vi "PopulateQuizArrayfromFile.vi"(8 "error in (no error)":errorcluster, 11 "file path (dialog if empty)":path) -> (0 "error out":errorcluster, 1 "Raw Data":string[][](array[string]), 2 "Question Array Out":T1[](array[typedef]))   [LabVIEW 2010]
uses:
  Controls/Quiz Set Up.ctl
  Controls/Problem Type enum.ctl
  Controls/Solution Type enum.ctl
  <vilib>/Utility/file.llb/Read From Spreadsheet File (string).vi
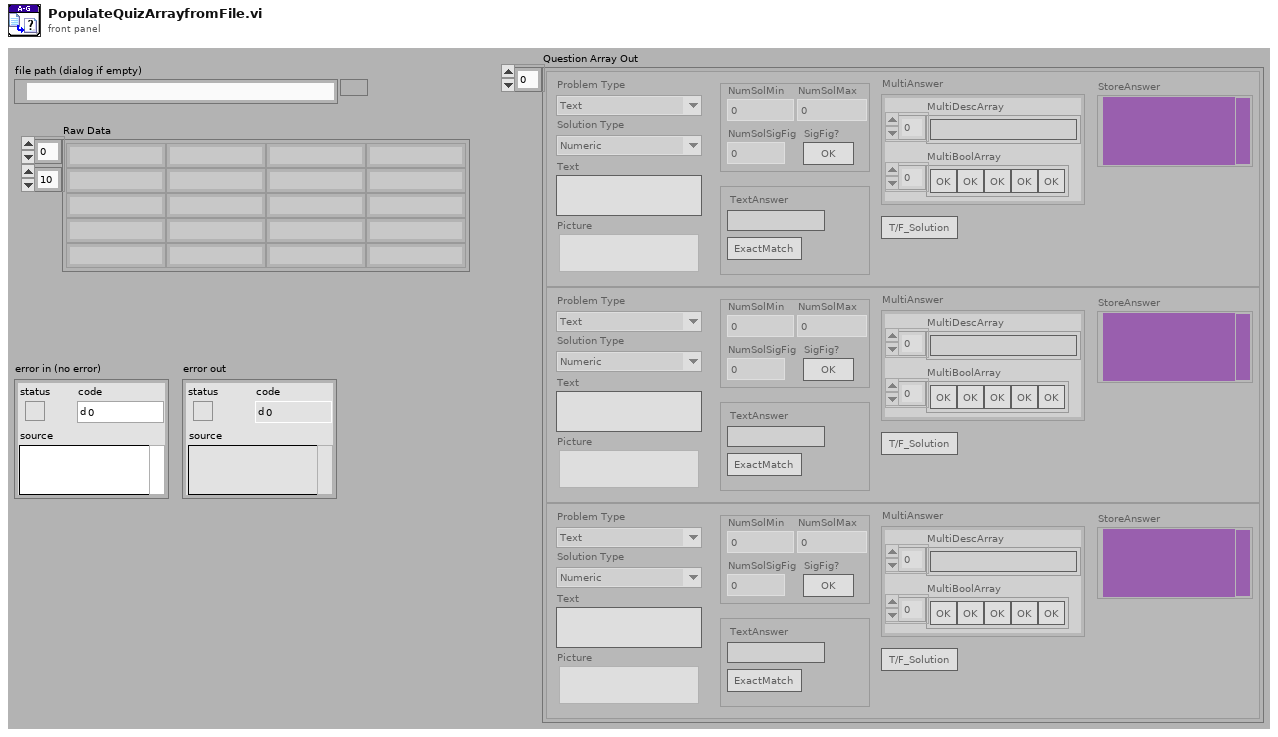
[diagram p1: front panel]
types:
  T1 = typedef "Quiz Set Up.ctl" = cluster{"Problem Type":T2, "Solution Type":T3, "Text":string, "Picture":picture, "NumSolMin":dbl, "NumSolMax":dbl, "SigFig?":bool, "NumSolSigFig":u32, "TextAnswer":string, "ExactMatch":bool, "T/F_Solution":bool, "StoreAnswer":variant, "MultiAnswer":cluster{"MultiDescArray":string[], "MultiBoolArray":bool[]}}
  T2 = typedef "Problem Type enum.ctl" = enum16{"Text", "Image", "Text&Image"}
  T3 = typedef "Solution Type enum.ctl" = enum16{"Numeric", "Text", "SelectMultiple", "SelectOne", "True/False", "ShortAnswer"}
  T4 = typedef "imagedata.ctl" = cluster{"image type":i32, "image depth":i32, "image":u8[], "mask":u8[], "colors":u32[], "Rectangle":cluster{"left":i16, "top":i16, "right":i16, "bottom":i16}}
  T5 = cluster{"MultiDescArray":string[], "MultiBoolArray":bool[]}
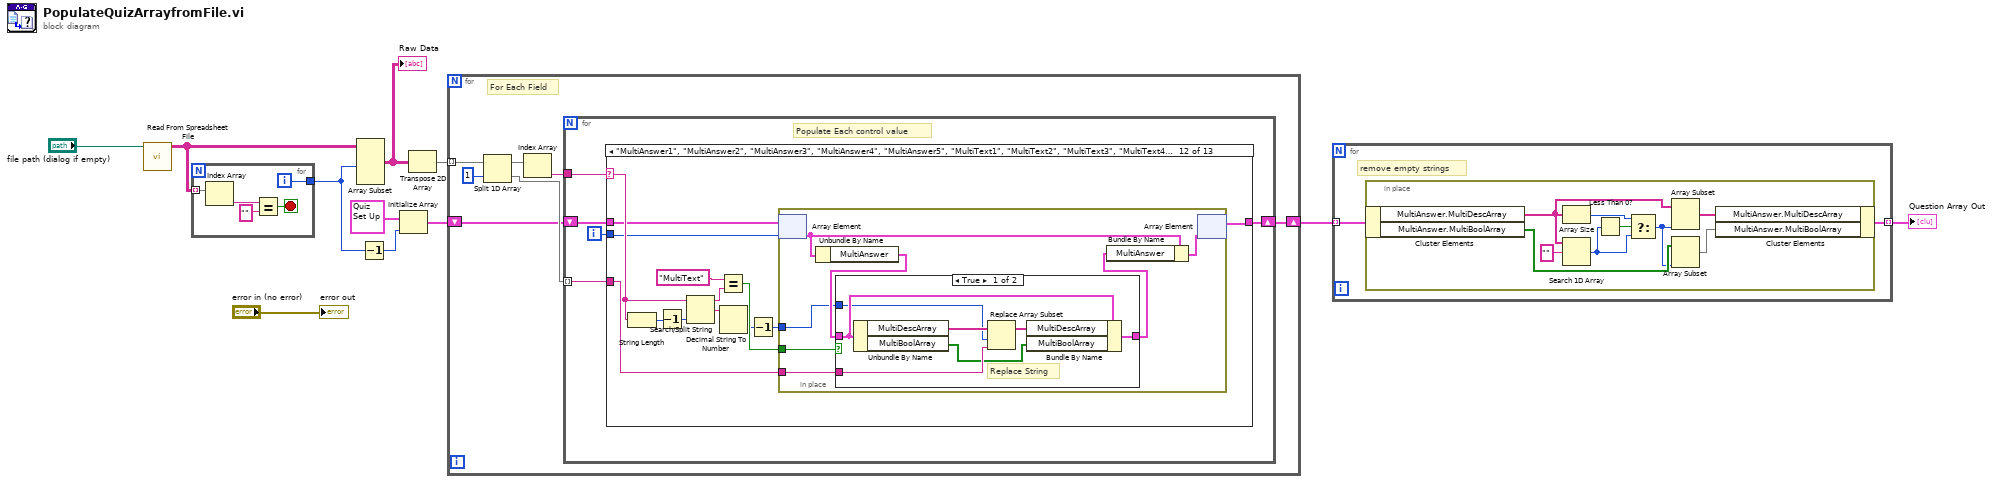
[diagram p0: block diagram]
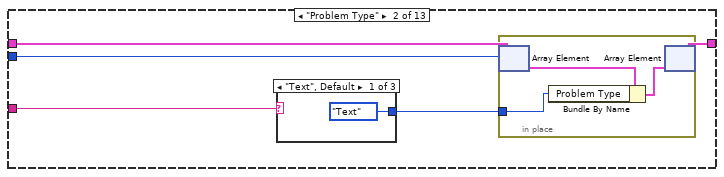
[diagram p3: hidden frame]
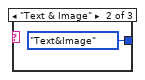
[diagram p4: hidden frame]
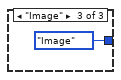
[diagram p5: hidden frame]
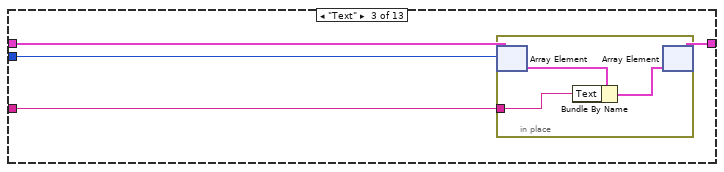
[diagram p6: hidden frame]
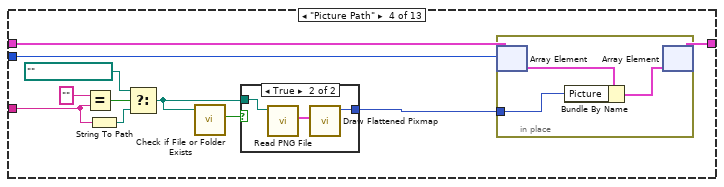
[diagram p7: hidden frame]
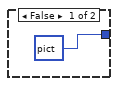
[diagram p8: hidden frame]
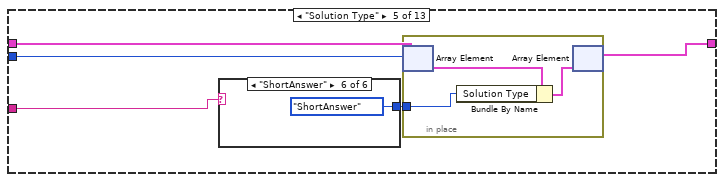
[diagram p9: hidden frame]
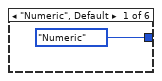
[diagram p10: hidden frame]
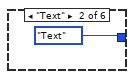
[diagram p11: hidden frame]
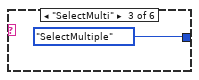
[diagram p12: hidden frame]
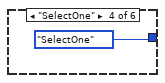
[diagram p13: hidden frame]
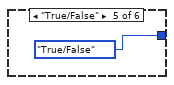
[diagram p14: hidden frame]
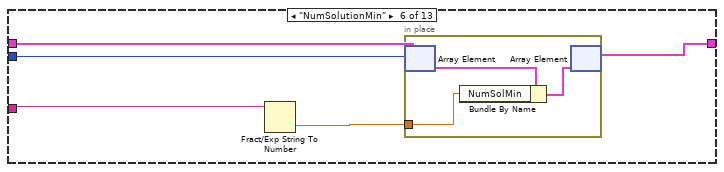
[diagram p15: hidden frame]
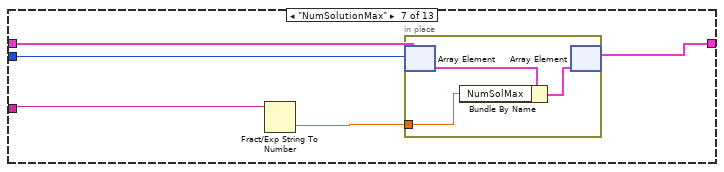
[diagram p16: hidden frame]
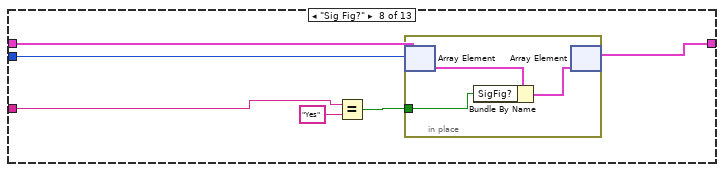
[diagram p17: hidden frame]
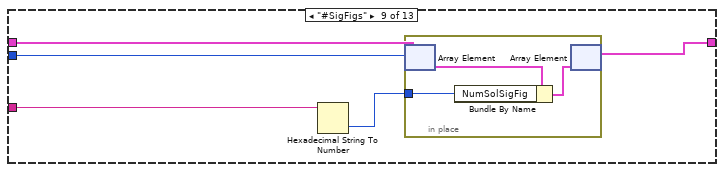
[diagram p18: hidden frame]
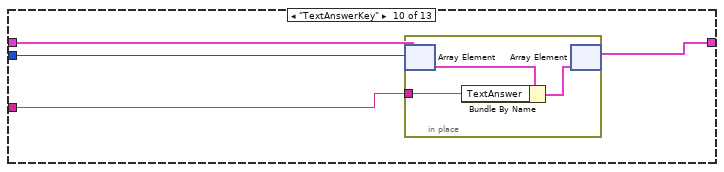
[diagram p19: hidden frame]
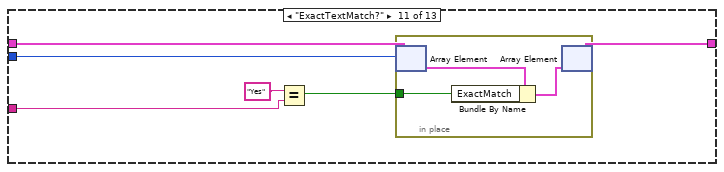
[diagram p20: hidden frame]
diagram:
  n1 = call-poly <vilib>:"Read From Spreadsheet File.vi"("file path (dialog if empty)"="file path (dialog if empty)") -> ("all rows"=w8:string[][])  [unwired: 6 in, 4 out]
  n2 = for {
    tunnel: [w15] -> w1
    tunnel: w8 -> [w14] mode=indexing
    i -> [w15]
    stop <- w12 stop-if-true
    n3 = Index Array(array=w14) -> (element=w13:string)  [unwired: 1 in]
    n4 = Equal?(x=w13, y="") -> (x = y?=w12:bool)
  }
  n5 = Array Subset(array=w8, length (row)=w1) -> (w9:string[][])  [unwired: 3 in]
  "Raw Data" <- w9
  n6 = Decrement(x=w1) -> (x-1=w2:i32)
  n7 = Initialize Array(T1 {"Problem Type"=enum."Text", "Solution Type"=enum."Numeric", "Text"="The sky is blue.", "Picture"=bytes[0], "NumSolMin"=0.0, "NumSolMax"=0.0, "SigFig?"=FALSE, "NumSolSigFig"=0, "TextAnswer"="", "ExactMatch"=FALSE, "T/F_Solution"=FALSE, "StoreAnswer"=variant, "MultiAnswer"={"MultiDescArray"=["", "", "", "", ""], "MultiBoolArray"=[FALSE, FALSE, FALSE, FALSE, FALSE]}} ("Quiz Set Up"), w2) -> (w5:T1[])
  n8 = Transpose 2D Array(2D array=w9) -> (transposed array=w11:string[][])
  n9 = for {
    tunnel: w11 -> [w23] mode=indexing
    shift-right: [w17] -> w3
    shift-left: w5 -> [w19]
    # "For Each Field"
    n10 = Split 1D Array(array=w23, index=1) -> (first subarray=w20:string[], second subarray=w21:string[])
    n11 = Index Array(array=w20) -> (element=w18:string)  [unwired: 1 in]
    n12 = for {
      tunnel: w21 -> [w28] mode=indexing
      tunnel: w18 -> [w27]
      shift-right: [w25] -> w17
      shift-left: w19 -> [w26]
      i -> [w24]
      # "Populate Each control value"
      n13 = case shown="\"MultiAnswer1\", \"MultiAnswer2\", \"MultiAnswer3\", \"MultiAnswer4\", \"MultiAnswer5\", \"MultiText1\", \"MultiText2\", \"MultiText3\", \"MultiText4\", \"MultiText5\"" w27 {
        selector: w27 -> [_ _ _ _ _ _ _ _ _ _ _ w136 _]
        tunnel: w28 -> [_ w34 w41 w53 w68 w84 w92 w98 w106 w113 w122 w130 w167]
        tunnel: w26 -> [w29 w33 w44 w57 w70 w82 w90 w100 w108 w115 w124 w135 w169]
        tunnel: [w29 w32 w43 w58 w69 w80 w88 w99 w107 w114 w125 w129 w170] -> w25
        tunnel: w24 -> [_ w30 w42 w55 w66 w83 w91 w101 w109 w116 w123 w134 w168]
        frame "NULL", Default {
        }
        frame "Problem Type" {
          n14 = case shown="\"Text\", Default" w34 {
            tunnel: [Problem_Type_enum."Text" ("Problem Type") Problem_Type_enum."Text&Image" ("Problem Type") Problem_Type_enum."Image" ("Problem Type")] -> w31
            frame "Text", Default {
            }
            frame "Text & Image" {
            }
            frame "Image" {
            }
          }
          n15 = in-place {
            in-place-border: w31 -> [w35]
            n16 = in-place-array #1(w33, w30) -> (w37:T1)
            n17 = Bundle By Name(cluster=w37, "Problem Type"=w35) -> (w36:T1)
            n18 = in-place-array #1(w36) -> (w32:T1[])  [unwired: 1 out]
          }
        }
        frame "Text" {
          n19 = in-place {
            in-place-border: w41 -> [w45]
            n20 = in-place-array #2(w44, w42) -> (w47:T1)
            n21 = Bundle By Name(cluster=w47, "Text"=w45) -> (w46:T1)
            n22 = in-place-array #2(w46) -> (w43:T1[])  [unwired: 1 out]
          }
        }
        frame "Picture Path" {
          n23 = Equal?(x="", y=w53) -> (x = y?=w51:bool)
          n24 = String To Path(string=w53) -> (path=w50:path)
          n25 = Select(t=path "", s=w51, f=w50) -> (s? t:f=w49:path)
          n26 = call <vilib>:"Check if File or Folder Exists.vi"("path"=w49) -> ("file or folder exists?"=w54:bool)  [unwired: 8 in, 2 out]
          n27 = case shown="True" w54 {
            tunnel: [picture data[5B] ("new picture") w61] -> w56
            tunnel: w49 -> [_ w60]
            frame False {
            }
            frame True {
              n28 = call <vilib>:"Read PNG File.vi"("path to PNG file"=w60) -> ("image data"=w62:T4)  [unwired: 8 in, 2 out]
              n29 = call <vilib>:"Draw Flattened Pixmap.vi"("image data"=w62) -> ("new picture"=w61:picture)  [unwired: 8 in]
            }
          }
          n30 = in-place {
            in-place-border: w56 -> [w63]
            n31 = in-place-array #3(w57, w55) -> (w65:T1)
            n32 = Bundle By Name(cluster=w65, "Picture"=w63) -> (w64:T1)
            n33 = in-place-array #3(w64) -> (w58:T1[])  [unwired: 1 out]
          }
        }
        frame "Solution Type" {
          n34 = case shown="\"ShortAnswer\"" w68 {
            tunnel: [Solution_Type_enum."Numeric" ("Solution Type") Solution_Type_enum."Text" ("Solution Type") Solution_Type_enum."SelectMultiple" ("Solution Type") Solution_Type_enum."SelectOne" ("Solution Type") Solution_Type_enum."True/False" ("Solution Type") Solution_Type_enum."ShortAnswer" ("Solution Type")] -> w67
            frame "Numeric", Default {
            }
            frame "Text" {
            }
            frame "SelectMulti" {
            }
            frame "SelectOne" {
            }
            frame "True/False" {
            }
            frame "ShortAnswer" {
            }
          }
          n35 = in-place {
            in-place-border: w67 -> [w77]
            n36 = in-place-array #4(w70, w66) -> (w79:T1)
            n37 = Bundle By Name(cluster=w79, "Solution Type"=w77) -> (w78:T1)
            n38 = in-place-array #4(w78) -> (w69:T1[])  [unwired: 1 out]
          }
        }
        frame "NumSolutionMin" {
          n39 = Fract/Exp String To Number(string=w84) -> (number=w81:dbl)  [unwired: 3 in, 1 out]
          n40 = in-place {
            in-place-border: w81 -> [w85]
            n41 = in-place-array #5(w82, w83) -> (w87:T1)
            n42 = Bundle By Name(cluster=w87, "NumSolMin"=w85) -> (w86:T1)
            n43 = in-place-array #5(w86) -> (w80:T1[])  [unwired: 1 out]
          }
        }
        frame "NumSolutionMax" {
          n44 = Fract/Exp String To Number(string=w92) -> (number=w89:dbl)  [unwired: 3 in, 1 out]
          n45 = in-place {
            in-place-border: w89 -> [w93]
            n46 = in-place-array #6(w90, w91) -> (w95:T1)
            n47 = Bundle By Name(cluster=w95, "NumSolMax"=w93) -> (w94:T1)
            n48 = in-place-array #6(w94) -> (w88:T1[])  [unwired: 1 out]
          }
        }
        frame "Sig Fig?" {
          n49 = Equal?(x=w98, y="Yes") -> (x = y?=w96:bool)
          n50 = in-place {
            in-place-border: w96 -> [w102]
            n51 = in-place-array #7(w100, w101) -> (w104:T1)
            n52 = Bundle By Name(cluster=w104, "SigFig?"=w102) -> (w103:T1)
            n53 = in-place-array #7(w103) -> (w99:T1[])  [unwired: 1 out]
          }
        }
        frame "#SigFigs" {
          n54 = Hexadecimal String To Number(string=w106) -> (number=w105:u32)  [unwired: 2 in, 1 out]
          n55 = in-place {
            in-place-border: w105 -> [w110]
            n56 = in-place-array #8(w108, w109) -> (w112:T1)
            n57 = Bundle By Name(cluster=w112, "NumSolSigFig"=w110) -> (w111:T1)
            n58 = in-place-array #8(w111) -> (w107:T1[])  [unwired: 1 out]
          }
        }
        frame "TextAnswerKey" {
          n59 = in-place {
            in-place-border: w113 -> [w117]
            n60 = in-place-array #9(w115, w116) -> (w119:T1)
            n61 = Bundle By Name(cluster=w119, "TextAnswer"=w117) -> (w118:T1)
            n62 = in-place-array #9(w118) -> (w114:T1[])  [unwired: 1 out]
          }
        }
        frame "ExactTextMatch?" {
          n63 = Equal?(x="Yes" ("y"), y=w122) -> (x = y?=w120:bool)
          n64 = in-place {
            in-place-border: w120 -> [w126]
            n65 = in-place-array #10(w124, w123) -> (w128:T1)
            n66 = Bundle By Name(cluster=w128, "ExactMatch"=w126) -> (w127:T1)
            n67 = in-place-array #10(w127) -> (w125:T1[])  [unwired: 1 out]
          }
        }
        frame "MultiAnswer1", "MultiAnswer2", "MultiAnswer3", "MultiAnswer4", "MultiAnswer5", "MultiText1", "MultiText2", "MultiText3", "MultiText4", "MultiText5" {
          n68 = String Length(string=w136) -> (length=w140:i32)
          n69 = Decrement(x=w140) -> (x-1=w139:i32)
          n70 = Search/Split String(string=w136, offset (0)=w139) -> (substring before match=w138:string, match + rest of string=w141:string)  [unwired: 1 in, 1 out]
          n71 = Equal?(x="MultiText" ("String"), y=w138) -> (x = y?=w133:bool)
          n72 = Decimal String To Number(string=w141) -> (number=w132:i32)  [unwired: 2 in, 1 out]
          n73 = Decrement(x=w132) -> (x-1=w131:i32)
          n74 = in-place {
            in-place-border: w133 -> [w144]
            in-place-border: w131 -> [w143]
            in-place-border: w130 -> [w142]
            n75 = in-place-array #11(w135, w134) -> (w147:T1)
            n76 = Unbundle By Name(w147) -> ("MultiAnswer"=w146:T5)
            n77 = case shown="True" w144 {
              tunnel: w146 -> [w154 w164]
              tunnel: [w152 w163] -> w145
              tunnel: w143 -> [w151 w159]
              tunnel: w142 -> [w150 w157]
              frame True {
                # "Replace String"
                n78 = Unbundle By Name(w154) -> ("MultiDescArray"=w155:string[], "MultiBoolArray"=w149:bool[])
                n79 = Replace Array Subset(array=w155, new element=w150, index=w151) -> (w153:string[])
                n80 = Bundle By Name(cluster=w154, "MultiDescArray"=w153, "MultiBoolArray"=w149) -> (w152:T5)
              }
              frame False {
                # "Replace Bool"
                n81 = Unbundle By Name(w164) -> ("MultiDescArray"=w162:string[], "MultiBoolArray"=w161:bool[])
                n82 = Equal?(x=w157, y="TRUE") -> (x = y?=w156:bool)
                n83 = Replace Array Subset(array=w161, new element=w156, index=w159) -> (w160:bool[])
                n84 = Bundle By Name(cluster=w164, "MultiDescArray"=w162, "MultiBoolArray"=w160) -> (w163:T5)
              }
            }
            n85 = Bundle By Name(cluster=w147, "MultiAnswer"=w145) -> (w148:T1)
            n86 = in-place-array #11(w148) -> (w129:T1[])  [unwired: 1 out]
          }
        }
        frame "T/F_Answer" {
          n87 = Equal?(x="TRUE" ("y"), y=w167) -> (x = y?=w165:bool)
          n88 = in-place {
            in-place-border: w165 -> [w171]
            n89 = in-place-array #12(w169, w168) -> (w173:T1)
            n90 = Bundle By Name(cluster=w173, "T/F_Solution"=w171) -> (w172:T1)
            n91 = in-place-array #12(w172) -> (w170:T1[])  [unwired: 1 out]
          }
        }
      }
    }
  }
  n92 = for {
    tunnel: w3 -> [w175] mode=indexing
    tunnel: [w174] -> w4 mode=indexing
    # "remove empty strings"
    n93 = in-place {
      n94 = in-place-cluster #13(w175) -> ("MultiAnswer.MultiDescArray"=w178:string[], "MultiAnswer.MultiBoolArray"=w182:bool[])
      n95 = Array Size(array=w178) -> (size(s)=w177:i32)
      n96 = Search 1D Array(1D array=w178, element="") -> (index of element=w179:i32)  [unwired: 1 in]
      n97 = Less Than 0?(x=w179) -> (x < 0?=w180:bool)
      n98 = Select(t=w177, s=w180, f=w179) -> (s? t:f=w176:i32)
      n99 = Array Subset(array=w178, length=w176) -> (w183:string[])  [unwired: 1 in]
      n100 = Array Subset(array=w182, length=w176) -> (w181:bool[])  [unwired: 1 in]
      n101 = in-place-cluster #13("MultiAnswer.MultiDescArray"=w183, "MultiAnswer.MultiBoolArray"=w181) -> (w174:T1)
    }
  }
  "Question Array Out" <- w4
  "error out" <- "error in (no error)"
